vi "AudioTest.Parse SoundCheck Results Item.vi"(10 "Name Lookup":variant, 11 "Result Record":string[](array[string])) -> (3 "Measurements":T1[](array[typedef]) {"Status" items=["LOG", "PASS", "FAIL", "ERROR"]})   [LabVIEW 2018]
uses:
  Common/Utils/Results/Result.Measurement Item.ctl
  Common/Utils/Results/Result.Measurement and Attribute Item Status.ctl
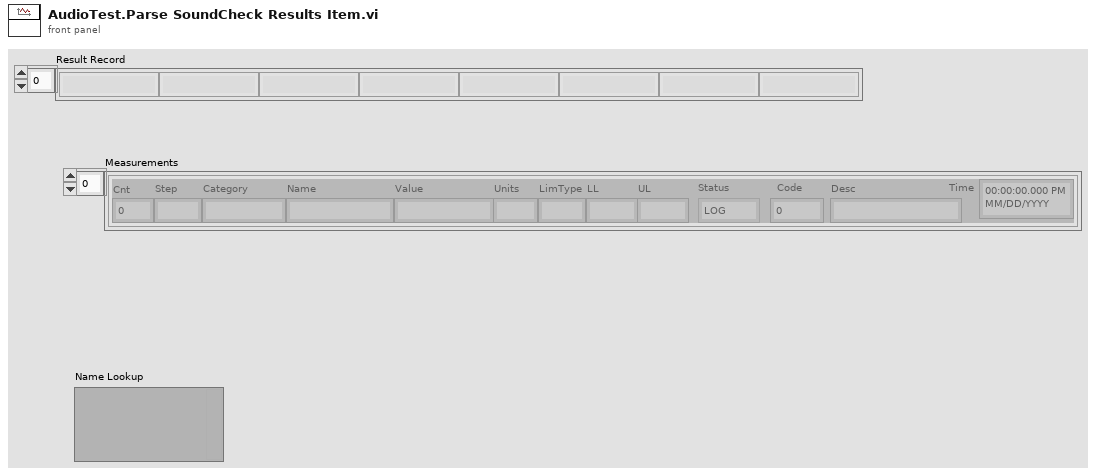
[diagram p1: front panel]
types:
  T1 = typedef "Result.Measurement Item.ctl" = cluster{"Cnt":i32, "Step":string, "Category":string, "Name":string, "Value":string, "Units":string, "LimType":string, "LL":string, "UL":string, "Status":T2, "Code":i32, "Desc":string, "Time":timestamp}
  T2 = typedef "Result.Measurement and Attribute Item Status.ctl" = i32
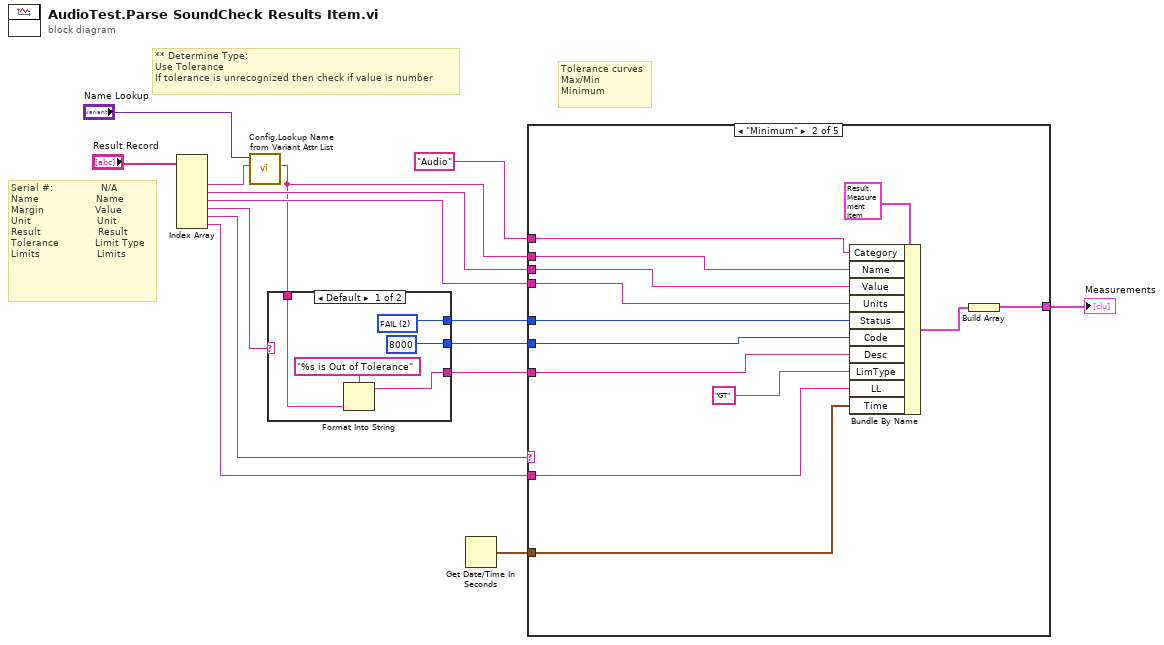
[diagram p0: block diagram]
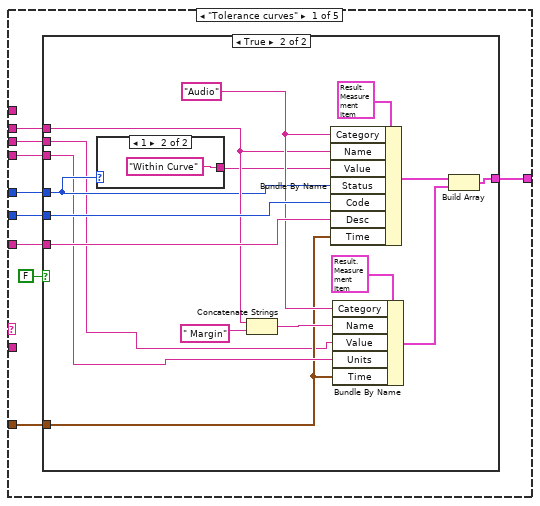
[diagram p2: hidden frame]
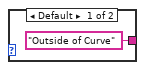
[diagram p4: hidden frame]
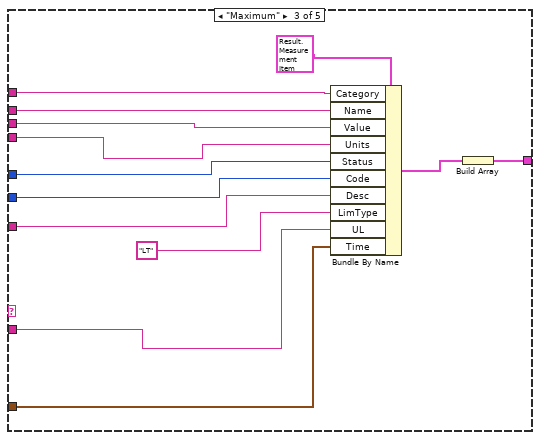
[diagram p5: hidden frame]
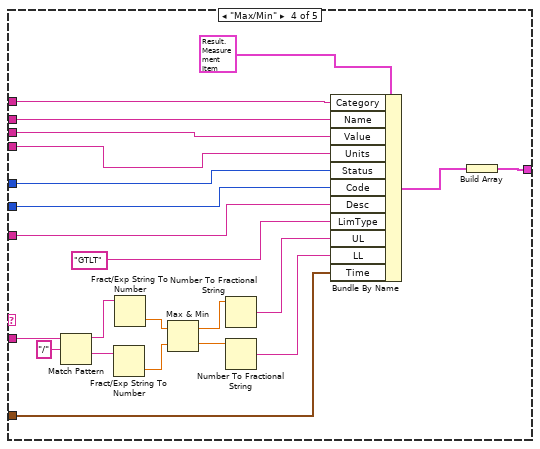
[diagram p6: hidden frame]
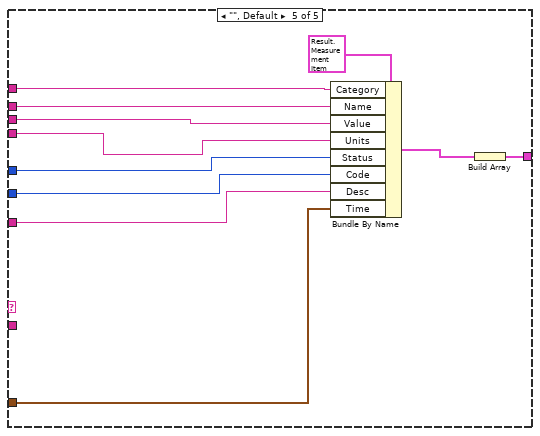
[diagram p7: hidden frame]
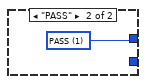
[diagram p8: hidden frame]
diagram:
  # "Serial #:\t               N/A\nName\t                  Name\nMargin\t                Value\nUnit\t                     Unit\nResult\t                  Result\nTolerance\t           Limit Type\nLimits\t                  Limits"
  # "** Determine Type:\nUse Tolerance\nIf tolerance is unrecognized then check if value is number"
  # "Tolerance curves\nMax/Min\nMinimum"
  n1 = Index Array(array="Result Record") -> (element #2=w2:string, element #3=w9:string, element #4=w10:string, element #5=w14:string, element #6=w8:string, element #7=w7:string)  [unwired: 7 in, 1 out]
  n2 = call "Config.Lookup Name from Variant Attr List.vi"("Name In"=w2, "Variant"="Name Lookup") -> ("Name Out"=w1:string)  [unwired: 9 in]
  n3 = case shown="Default" w14 {
    tunnel: [w20 w21] -> w13
    tunnel: [8000 _] -> w12
    tunnel: [w17 _] -> w11
    tunnel: w1 -> [w16 _]
    frame Default {
      w20 = T2 2 items=["LOG", "PASS", "FAIL", "ERROR"] ("Status")
      n4 = Format Into String(format string="%s is Out of Tolerance", w16) -> (resulting string=w17:string)  [unwired: 2 in, 1 out]
    }
    frame "PASS" {
      w21 = T2 1 items=["LOG", "PASS", "FAIL", "ERROR"] ("Status")
    }
  }
  n5 = Get Date/Time In Seconds() -> (seconds since 1Jan1904=w4:timestamp)
  n6 = case shown="\"Minimum\"" w8 {
    tunnel: w1 -> [w27 w61 w74 w96 w107]
    tunnel: w9 -> [w25 w52 w65 w80 w98]
    tunnel: w10 -> [w24 w60 w73 w95 w106]
    tunnel: w13 -> [w26 w59 w72 w94 w105]
    tunnel: w12 -> [w30 w58 w71 w93 w104]
    tunnel: w11 -> [w29 w57 w70 w92 w103]
    tunnel: [w28 w49 w62 w75 w97] -> w5
    tunnel: w7 -> [_ w51 w63 w88 _]
    tunnel: "Audio" ("Category") -> [_ w55 w68 w90 w101]
    tunnel: w4 -> [w23 w54 w67 w89 w100]
    frame "Tolerance curves" {
      n7 = case shown="True" FALSE {
        tunnel: w30 -> [_ w46]
        tunnel: w29 -> [_ w45]
        tunnel: [_ w43] -> w28
        tunnel: w27 -> [_ w40]
        tunnel: w26 -> [_ w38]
        tunnel: w25 -> [_ w32]
        tunnel: w24 -> [_ w36]
        tunnel: w23 -> [_ w35]
        frame False {
        }
        frame True {
          w42 = "Audio" ("Category")
          n8 = case shown="1" w38 {
            tunnel: ["Outside of Curve" "Within Curve"] -> w37
            frame Default {
            }
            frame 1 {
            }
          }
          n9 = Concatenate Strings(w40, " Margin") -> (w39:string)
          n10 = Bundle By Name(cluster=T1 {"Cnt"=0, "Step"="", "Category"="", "Name"="", "Value"="", "Units"="", "LimType"="", "LL"="", "UL"="", "Status"=0, "Code"=0, "Desc"="", "Time"=timestamp(0 s since 1904-01-01)} ("Meas"), "Category"=w42, "Name"=w40, "Value"=w37, "Status"=w38, "Code"=w46, "Desc"=w45, "Time"=w35) -> (w44:T1)
          n11 = Bundle By Name(cluster=T1 {"Cnt"=0, "Step"="", "Category"="", "Name"="", "Value"="", "Units"="", "LimType"="", "LL"="", "UL"="", "Status"=0, "Code"=0, "Desc"="", "Time"=timestamp(0 s since 1904-01-01)} ("Meas"), "Category"=w42, "Name"=w39, "Value"=w32, "Units"=w36, "Time"=w35) -> (w31:T1)
          n12 = Build Array(w44, w31) -> (w43:T1[])
        }
      }
    }
    frame "Minimum" {
      n13 = Bundle By Name(cluster=T1 {"Cnt"=0, "Step"="", "Category"="", "Name"="", "Value"="", "Units"="", "LimType"="", "LL"="", "UL"="", "Status"=0, "Code"=0, "Desc"="", "Time"=timestamp(0 s since 1904-01-01)} ("Meas"), "Category"=w55, "Name"=w61, "Value"=w52, "Units"=w60, "Status"=w59, "Code"=w58, "Desc"=w57, "LimType"="GT", "LL"=w51, "Time"=w54) -> (w56:T1)
      n14 = Build Array(w56) -> (w49:T1[])
    }
    frame "Maximum" {
      n15 = Bundle By Name(cluster=T1 {"Cnt"=0, "Step"="", "Category"="", "Name"="", "Value"="", "Units"="", "LimType"="", "LL"="", "UL"="", "Status"=0, "Code"=0, "Desc"="", "Time"=timestamp(0 s since 1904-01-01)} ("Meas"), "Category"=w68, "Name"=w74, "Value"=w65, "Units"=w73, "Status"=w72, "Code"=w71, "Desc"=w70, "LimType"="LT", "UL"=w63, "Time"=w67) -> (w69:T1)
      n16 = Build Array(w69) -> (w62:T1[])
    }
    frame "Max/Min" {
      n17 = Match Pattern(string=w88, regular expression="/") -> (before substring=w86:string, after substring=w85:string)  [unwired: 1 in, 2 out]
      n18 = Fract/Exp String To Number(string=w85) -> (number=w83:dbl)  [unwired: 3 in, 1 out]
      n19 = Fract/Exp String To Number(string=w86) -> (number=w84:dbl)  [unwired: 3 in, 1 out]
      n20 = Max & Min(x=w84, y=w83) -> (max(x,y)=w79:dbl, min(x,y)=w78:dbl)
      n21 = Number To Fractional String(number=w79) -> (F-format string=w76:string)  [unwired: 3 in]
      n22 = Number To Fractional String(number=w78) -> (F-format string=w77:string)  [unwired: 3 in]
      n23 = Bundle By Name(cluster=T1 {"Cnt"=0, "Step"="", "Category"="", "Name"="", "Value"="", "Units"="", "LimType"="", "LL"="", "UL"="", "Status"=0, "Code"=0, "Desc"="", "Time"=timestamp(0 s since 1904-01-01)} ("Meas"), "Category"=w90, "Name"=w96, "Value"=w80, "Units"=w95, "Status"=w94, "Code"=w93, "Desc"=w92, "LimType"="GTLT", "UL"=w76, "LL"=w77, "Time"=w89) -> (w91:T1)
      n24 = Build Array(w91) -> (w75:T1[])
    }
    frame "", Default {
      n25 = Bundle By Name(cluster=T1 {"Cnt"=0, "Step"="", "Category"="", "Name"="", "Value"="", "Units"="", "LimType"="", "LL"="", "UL"="", "Status"=0, "Code"=0, "Desc"="", "Time"=timestamp(0 s since 1904-01-01)} ("Meas"), "Category"=w101, "Name"=w107, "Value"=w98, "Units"=w106, "Status"=w105, "Code"=w104, "Desc"=w103, "Time"=w100) -> (w102:T1)
      n26 = Build Array(w102) -> (w97:T1[])
    }
  }
  "Measurements" <- w5
